vi "SUB_COM1_ESC3.vi"   [LabVIEW 2011]
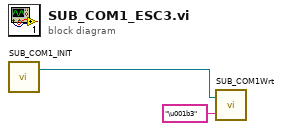
[diagram p0: block diagram]
diagram:
  n1 = call "SUB_COM1_INIT.vi"() -> ("VISA resource name out"=w2:refnum<visa-resource-name>)  [unwired: 2 in, 1 out]
  n2 = call "SUB_COM1Wrt.vi"("VISA resource name"=w2, "write buffer"="\u001b3") -> ()  [unwired: 3 out]
